vi "LVClass_Camera ctor Instance.vi"(0 "Camera (const)":refnum<class "Camera.lvclass">, 5 "Configuration file path":path, 11 "error in (no error)":errorcluster) -> (4 "Camera (new)":refnum<class "Camera.lvclass">, 15 "error out":errorcluster)   [LabVIEW 2020, in "Camera.lvclass"]
doc: "Camera instance constructor.\n\n<B>CameraIn</B> : Constant Pointer to Camera object.\n<B>CameraOut</B> : Constant Pointer to Camera object.\n<B>config_file_path</B> : Absolute path to Haso or Camera configuration file."
uses:
  Camera.lvclass
  Handle creation.ctl
  Camera.lvclass/Camera.ctl
  CameraSet.lvclass
  Image.lvclass
  Data alignment enum.ctl
  CameraAcquisitionState.ctl
  LVClass_CameraSet Read CameraParameters.vi
  LVClass_CameraSet Read AllValueSetAndGet.vi
  LVClass_CameraSet Read AllValueGet.vi
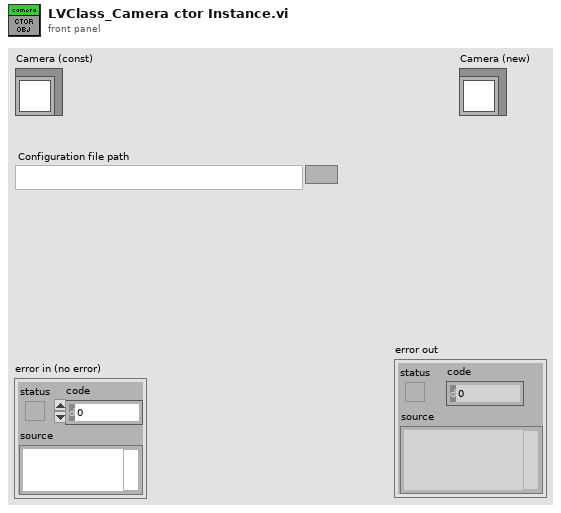
[diagram p1: front panel]
types:
  T1 = typedef "Handle creation.ctl" = enum16{"By ctor", "By write function"}
  T2 = typedef "Data alignment enum.ctl" = enum16{"8", "16", "32"}
  T3 = typedef "CameraAcquisitionState.ctl" = enum16{"Stop", "Live"}
  T4 = typedef "ParameterID.ctl" = cluster{"Name":string, "ConnectionParameter?":bool, "Type":T5, "Authorization":T6, "OnFlyAuthorization":T7, "StringValue":string, "Value":dbl, "Min":dbl, "Max":dbl, "BooleanValue":bool, "StringParameterList":string[]}
  T5 = typedef "CameraParameters_Type.ctl" = enum16{"Integer", "Real", "String", "Boolean"}
  T6 = typedef "CameraParameters_Authorization.ctl" = enum16{"Disable", "Gettable", "Settable - Gettable"}
  T7 = typedef "CameraParameters_OnFlyAuthorization.ctl" = enum16{"None", "Gettable", "Settable", "Settable - Gettable"}
  T8 = typedef "CameraParametersSetup.ctl" = cluster{"Name":string, "Type":T5, "Value":dbl, "BooleanValue":bool, "StringValue":string, "ConnectionParameter":bool}
  T9 = typedef "CameraSpecifications.ctl" = cluster{"Grabber name":string, "Camera name":string, "Camera sn":string, "Pixels_um":T10, "Maximum level":u32, "Data alignment":T2, "Is signed":bool, "Acquisition start":T11, "Acquisition length":T11, "MaxFrameRate_Hz":sgl, "Chip type":enum16{"Progressive scan", "Frame transfert"}}
  T10 = typedef "General dimensions definition.ctl" = cluster{"Size":T11, "Step":T12}
  T11 = typedef "Point2D.ctl" = cluster{"X":u32, "Y":u32}
  T12 = typedef "Point2Df.ctl" = cluster{"X":sgl, "Y":sgl}
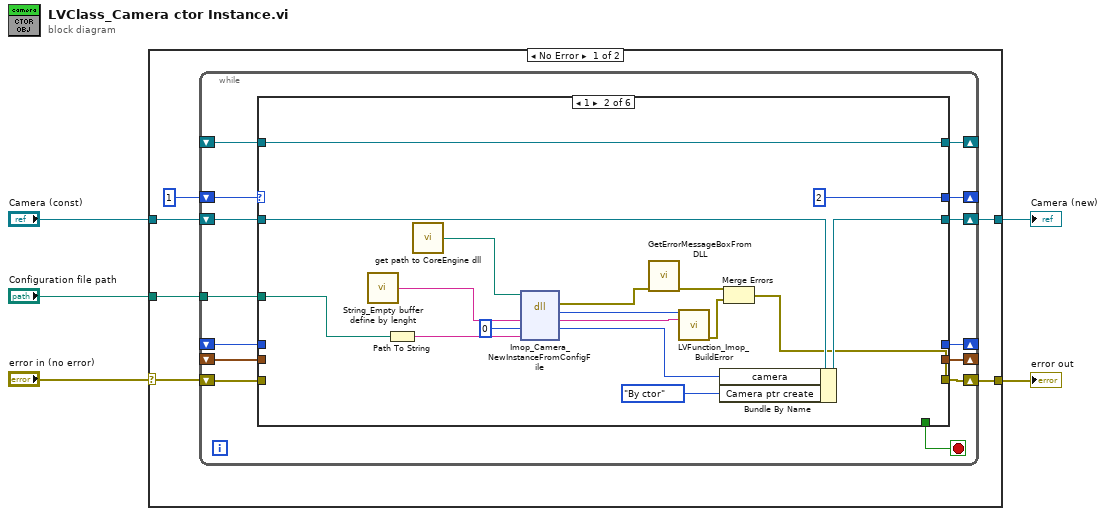
[diagram p0: block diagram]
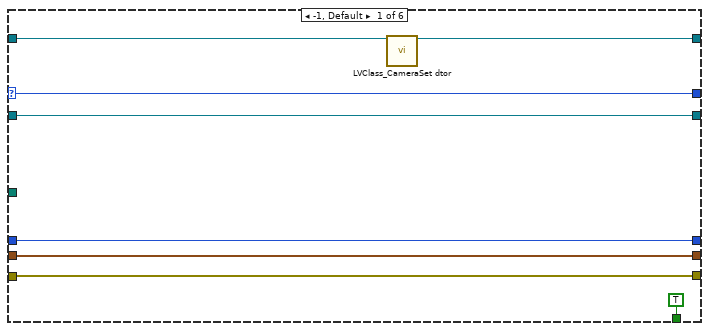
[diagram p2: hidden frame]
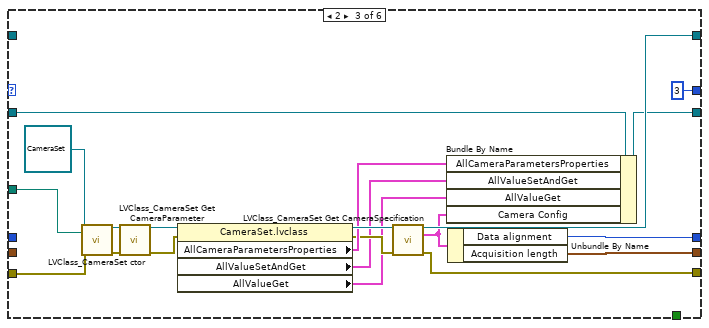
[diagram p3: hidden frame]
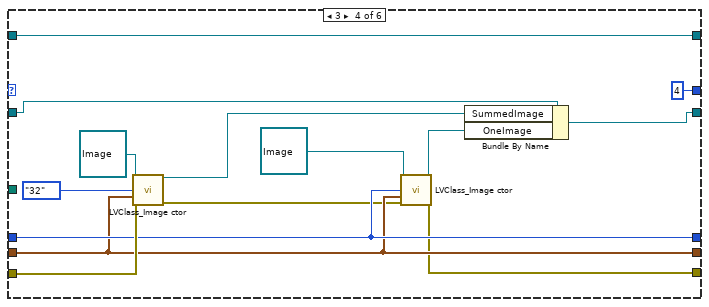
[diagram p4: hidden frame]
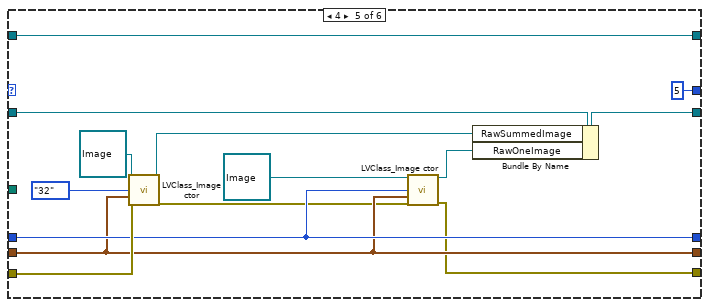
[diagram p5: hidden frame]
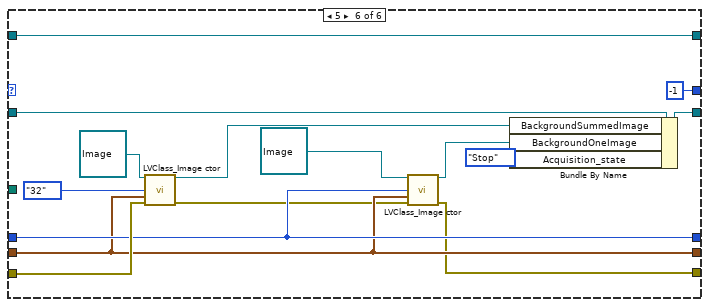
[diagram p6: hidden frame]
diagram:
  n1 = case shown="No Error" "error in (no error)" {
    selector: "error in (no error)" -> [w7 w115]
    tunnel: [w6 w115] -> w4
    tunnel: [w10 w114] -> w2
    tunnel: "Camera (const)" -> [w11 w114]
    tunnel: "Configuration file path" -> [w8 _]
    frame No Error {
      n2 = while {
        shift-right: [w23] -> _
        shift-left: 1 -> [w22]
        tunnel: w8 -> [w21]
        shift-right: [w20] -> w6
        shift-left: w7 -> [w19]
        shift-right: [w17] -> _
        shift-left: _ -> [w15]
        shift-right: [w18] -> _
        shift-left: _ -> [w16]
        shift-right: [w24] -> w10
        shift-left: w11 -> [w25]
        shift-right: [w13] -> _
        shift-left: _ -> [w12]
        stop <- w14 stop-if-true
        n3 = case shown="1" w22 {
          selector: w22 -> [w32 _ _ _ _ _]
          tunnel: [w31 w34 w66 w74 w88 w103] -> w20
          tunnel: w25 -> [w28 w45 w60 w82 w96 w111]
          tunnel: [w28 w44 w59 w81 w95 w110] -> w24
          tunnel: [w32 2 3 4 5 -1] -> w23
          tunnel: w21 -> [_ w39 w69 _ _ _]
          tunnel: w19 -> [w31 _ w68 w83 w97 w112]
          tunnel: [w29 _ w64 w78 w92 w107] -> w18
          tunnel: [w30 _ w67 w77 w91 w106] -> w17
          tunnel: w16 -> [w29 _ _ w78 w92 w107]
          tunnel: w15 -> [w30 _ _ w77 w91 w106]
          tunnel: [TRUE _ _ _ _ _] -> w14
          tunnel: [w26 w37 w63 w72 w86 w101] -> w13
          tunnel: w12 -> [w27 w37 _ w72 w86 w101]
          frame -1, Default {
            n4 = call "LVClass_CameraSet dtor.vi"("CameraSet in"=w27) -> ("CameraSet out"=w26:refnum<class "CameraSet.lvclass">)  [unwired: 13 in, 1 out]
          }
          frame 1 {
            n5 = call "String_Empty buffer define by lenght.vi"() -> ("Empty buffer"=w43:string)  [unwired: 1 in]
            n6 = Path To String(path=w39) -> (string=w38:string)
            n7 = call "get path to CoreEngine dll.vi"() -> ("path to c_interface_vc100.dll"=w42:path)  [unwired: 12 in, 3 out]
            n8 = dll-call lib="D:/soft/HASO_v3/SVN_trunk/ImOpCoreEngine4_LV2011/DLLs/c_interface_vc100.dll" fn="Imop_Camera_NewInstanceFromConfigFile"(path in=w42, "message"=w43, "objet"=0, "chemin_config"=w38) -> (error out=w41:errorcluster, "return type"=w48:i32, "message"=w47:string, "objet"=w46:i64)  [unwired: 3 in, 1 out]
            n9 = call "GetErrorMessageBoxFromDLL.vi"("error IN"=w41) -> ("error OUT"=w36:errorcluster)  [unwired: 10 in]
            n10 = call "LVFunction_Imop_BuildError.vi"("code"=w48, "String to Prepend to source (\"\")"=w47) -> ("error out"=w35:errorcluster)  [unwired: 13 in]
            n11 = Bundle By Name(cluster=w45, "camera"=w46, "Camera ptr create"=Handle_creation."By ctor" ("Haso ptr create")) -> (w44:refnum<class "Camera.lvclass">)
            n12 = Merge Errors(w36, w35) -> (w34:errorcluster)
          }
          frame 2 {
            n13 = call "LVClass_CameraSet ctor.vi"("CameraSet (const)"=refnum<class "CameraSet.lvclass"> refnum ("CameraSet.lvclass"), "Configuration file path"=w69, "error in (no error)"=w68) -> ("CameraSet (new)"=w62:refnum<class "CameraSet.lvclass">, "error out"=w61:errorcluster)  [unwired: 11 in]
            n14 = call "LVClass_CameraSet Get CameraParameter.vi"("CameraSet in"=w62, "error in (no error)"=w61) -> ("CameraSet out"=w58:refnum<class "CameraSet.lvclass">, "error out"=w56:errorcluster)  [unwired: 10 in, 2 out]
            n15 = property class="CameraSet.lvclass"(reference=w58, error in=w56) -> (reference out=w57:refnum<class "CameraSet.lvclass">, error out=w54:errorcluster, "AllCameraParametersProperties"=w55:T4[], "AllValueSetAndGet"=w53:T8[], "AllValueGet"=w51:T8[])
            n16 = call "LVClass_CameraSet Get CameraSpecification.vi"("CameraSet in"=w57, "error in (no error)"=w54) -> ("CameraSet out"=w63:refnum<class "CameraSet.lvclass">, "Camera Config"=w52:T9, "error out"=w66:errorcluster)  [unwired: 11 in]
            n17 = Bundle By Name(cluster=w60, "AllCameraParametersProperties"=w55, "AllValueSetAndGet"=w53, "AllValueGet"=w51, "Camera Config"=w52) -> (w59:refnum<class "Camera.lvclass">)
            n18 = Unbundle By Name(w52) -> ("Data alignment"=w64:T2, "Acquisition length"=w67:T11)
          }
          frame 3 {
            n19 = call "LVClass_Image ctor.vi"("Image (const)"=refnum<class "Image.lvclass"> refnum ("Image in"), "Data alignment"=Data_alignment_enum."32", "Size"=w77, "error in (no error)"=w83) -> ("Image (new)"=w80:refnum<class "Image.lvclass">, "error out"=w75:errorcluster)  [unwired: 10 in]
            n20 = call "LVClass_Image ctor.vi"("Image (const)"=refnum<class "Image.lvclass"> refnum ("Image in"), "Data alignment"=w78, "Size"=w77, "error in (no error)"=w75) -> ("Image (new)"=w76:refnum<class "Image.lvclass">, "error out"=w74:errorcluster)  [unwired: 10 in]
            n21 = Bundle By Name(cluster=w82, "SummedImage"=w80, "OneImage"=w76) -> (w81:refnum<class "Camera.lvclass">)
          }
          frame 4 {
            n22 = call "LVClass_Image ctor.vi"("Image (const)"=refnum<class "Image.lvclass"> refnum ("Image in"), "Data alignment"=Data_alignment_enum."32", "Size"=w91, "error in (no error)"=w97) -> ("Image (new)"=w94:refnum<class "Image.lvclass">, "error out"=w89:errorcluster)  [unwired: 10 in]
            n23 = call "LVClass_Image ctor.vi"("Image (const)"=refnum<class "Image.lvclass"> refnum ("Image in"), "Data alignment"=w92, "Size"=w91, "error in (no error)"=w89) -> ("Image (new)"=w90:refnum<class "Image.lvclass">, "error out"=w88:errorcluster)  [unwired: 10 in]
            n24 = Bundle By Name(cluster=w96, "RawSummedImage"=w94, "RawOneImage"=w90) -> (w95:refnum<class "Camera.lvclass">)
          }
          frame 5 {
            n25 = call "LVClass_Image ctor.vi"("Image (const)"=refnum<class "Image.lvclass"> refnum ("Image in"), "Data alignment"=Data_alignment_enum."32", "Size"=w106, "error in (no error)"=w112) -> ("Image (new)"=w109:refnum<class "Image.lvclass">, "error out"=w104:errorcluster)  [unwired: 10 in]
            n26 = call "LVClass_Image ctor.vi"("Image (const)"=refnum<class "Image.lvclass"> refnum ("Image in"), "Data alignment"=w107, "Size"=w106, "error in (no error)"=w104) -> ("Image (new)"=w105:refnum<class "Image.lvclass">, "error out"=w103:errorcluster)  [unwired: 10 in]
            n27 = Bundle By Name(cluster=w111, "BackgroundSummedImage"=w109, "BackgroundOneImage"=w105, "Acquisition_state"=CameraAcquisitionState."Stop") -> (w110:refnum<class "Camera.lvclass">)
          }
        }
      }
    }
    frame Error {
    }
  }
  "error out" <- w4
  "Camera (new)" <- w2
